vi "LVtoJSON-DBUpdateAll.vi"(4 "Datatype":i32, 5 "Column Number":i32, 6 "Payload":string="Inventory", 7 "Update All":bool, 8 "error in":errorcluster, 9 "Reply Command":string="Inventory", 10 "SQL Statement":string, 11 "Table":string="Inventory") -> (0 "error out":errorcluster, 3 "Output JSON Object":string)   [LabVIEW 2013]
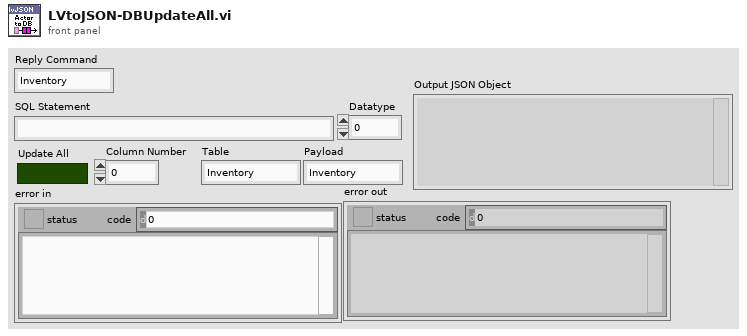
[diagram p1: front panel]
types:
  T1 = cluster{"Table":string, "SQL Statement":string, "Update All":bool, "Payload":string, "Column Number":i32, "Datatype":i32, "Reply Command":string}
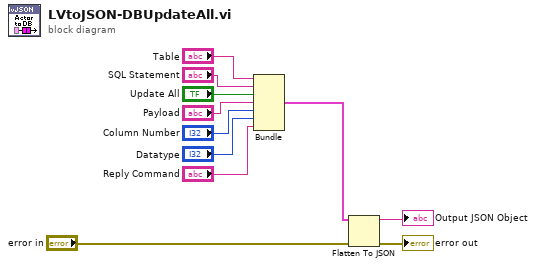
[diagram p0: block diagram]
diagram:
  n1 = Bundle("Table"="Table", "SQL Statement"="SQL Statement", "Update All"="Update All", "Payload"="Payload", "Column Number"="Column Number", "Datatype"="Datatype", "Reply Command"="Reply Command") -> (w5:T1)  [unwired: 1 in]
  n2 = Flatten To JSON(anything=w5, error in (no error)="error in") -> (JSON string=→"Output JSON Object":string, 11:→"error out":errorcluster)  [unwired: 1 in]
